vi "Write Distance to Plate Measured.vi"(10 "Distance to Plate Measured":dbl[unit]=1.0 min=1.0 max=300.0 format="%.1f", 11 "StiffnessMonitor in":refnum<class "StiffnessMonitor.lvclass">) -> (3 "StiffnessMonitor out":refnum<class "StiffnessMonitor.lvclass">)   [LabVIEW 2013, in "StiffnessMonitor.lvclass"]
uses:
  StiffnessMonitor.lvclass
  StiffnessMonitor.lvclass/StiffnessMonitor.ctl
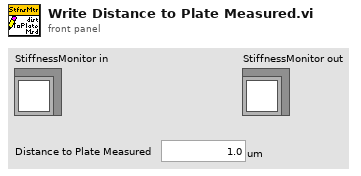
[diagram p1: front panel]
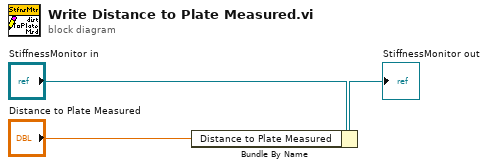
[diagram p0: block diagram]
diagram:
  n1 = Bundle By Name(cluster="StiffnessMonitor in", "Distance to Plate Measured"="Distance to Plate Measured") -> (→"StiffnessMonitor out":refnum<class "StiffnessMonitor.lvclass">)
